vi "Main.vi"() -> ()   [LabVIEW 2010]
uses:
  Ch1.ctl
  <vilib>/DAQmx/create/channels.llb/DAQmx Create Channel (AI-Voltage-Basic).vi
  <vilib>/DAQmx/read.llb/DAQmx Read (Analog DBL 1Chan 1Samp).vi
panel:
  out "Датчик Холла":dbl(graph)
  out "В, мТл":dbl format="%0.2f"
  in  "Exit":bool
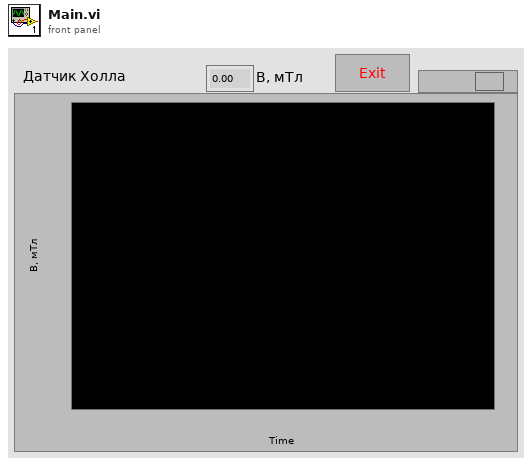
[diagram p1: front panel]
types:
  T1 = typedef "Ch1.ctl" = enum16{"def", "Exit", "A1", "P0"}
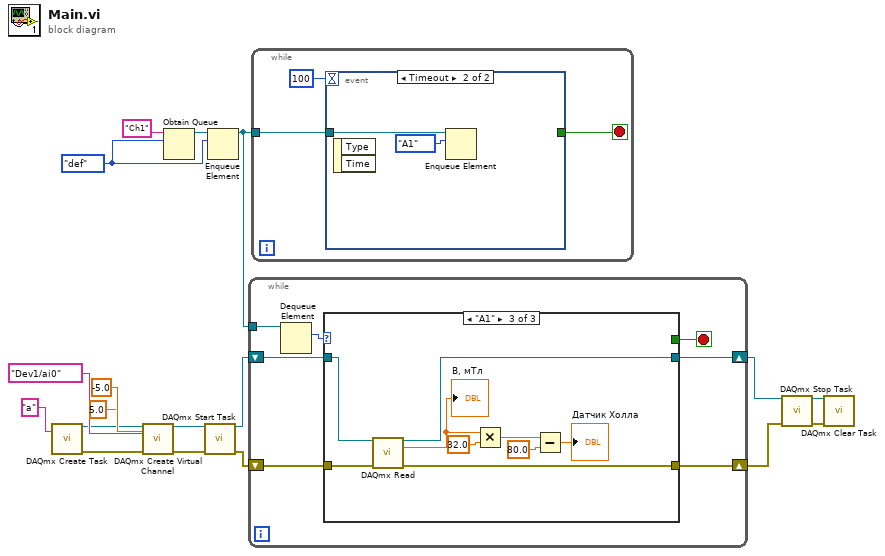
[diagram p0: block diagram]
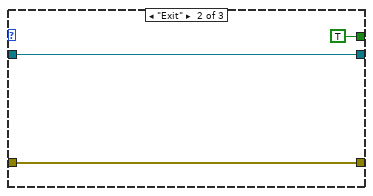
[diagram p3: hidden frame]
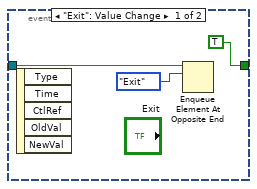
[diagram p4: hidden frame]
diagram:
  w18 = Ch1."def" ("Enum")
  n1 = call <vilib>:"DAQmx Create Task.vi"("new task name"="a") -> ("task out"=w6:refnum<k21>, "error out"=w5:errorcluster)  [unwired: 13 in]
  n2 = call-poly <vilib>:"DAQmx Create Virtual Channel.vi"("task in"=w6, "maximum value"=5.0, "minimum value"=-5.0, "physical channels"=tag "Dev1/ai0", "error in"=w5) -> ("task out"=w13:refnum<k21>, "error out"=w14:errorcluster)  [unwired: 9 in]
  n3 = Obtain Queue(name (unnamed)="Ch1", element data type=w18) -> (queue out=w17:refnum<queue>)  [unwired: 3 in, 2 out]
  n4 = call <vilib>:"DAQmx Start Task.vi"("task/channels in"=w13, "error in"=w14) -> ("task out"=w4:refnum<k21>, "error out"=w3:errorcluster)  [unwired: 12 in]
  n5 = Enqueue Element(queue=w17, element=w18) -> (queue out=w1:refnum<queue>)  [unwired: 2 in, 2 out]
  n6 = while {
    tunnel: w1 -> [w25]
    shift-right: [w19] -> w2
    shift-left: w3 -> [w20]
    shift-right: [w22] -> w7
    shift-left: w4 -> [w21]
    stop <- w23 stop-if-true
    n7 = Dequeue Element(queue=w25) -> (element=w24:T1)  [unwired: 2 in, 3 out]
    n8 = case shown="\"A1\"" w24 {
      tunnel: [_ TRUE _] -> w23
      tunnel: [w27 w29 w39] -> w22
      tunnel: w21 -> [w27 w29 w38]
      tunnel: w20 -> [w26 w28 w37]
      tunnel: [w26 w28 w36] -> w19
      frame "def", Default {
      }
      frame "Exit" {
      }
      frame "A1" {
        n9 = call-poly <vilib>:"DAQmx Read.vi"("task/channels in"=w38, "error in"=w37) -> ("task out"=w39:refnum<k21>, "data"=w31:dbl, "error out"=w36:errorcluster)  [unwired: 11 in]
        "В, мТл" <- w31
        n10 = Multiply(x=w31, y=32.0) -> (x*y=w34:dbl)
        n11 = Subtract(x=w34, y=80.0) -> (x-y=→"Датчик Холла":dbl)
      }
    }
  }
  n12 = while {
    tunnel: w1 -> [w42]
    stop <- w41 stop-if-true
    n13 = event shown="[1] Timeout" {
      selector: _ -> [_ _]
      dyn-events: _ -> [_ _]
      timeout: 100 -> [_ _]
      tunnel: w42 -> [w45 w47]
      tunnel: [TRUE _] -> w41
      event "Exit": Value Change {
        n14 = event-data() -> ()  [unwired: 1 in, 5 out]
        n15 = Enqueue Element At Opposite End(queue=w45, element=Ch1."Exit" ("Enum")) -> ()  [unwired: 2 in, 3 out]
      }
      event Timeout {
        n16 = event-data() -> ()  [unwired: 1 in, 2 out]
        n17 = Enqueue Element(queue=w47, element=Ch1."A1" ("Enum")) -> ()  [unwired: 2 in, 3 out]
      }
    }
  }
  n18 = call <vilib>:"DAQmx Stop Task.vi"("task/channels in"=w7, "error in"=w2) -> ("task out"=w9:refnum<k21>, "error out"=w8:errorcluster)  [unwired: 12 in]
  n19 = call <vilib>:"DAQmx Clear Task.vi"("task in"=w9, "error in"=w8) -> ()  [unwired: 13 in, 1 out]
